vi "FTW-CSV-Variant-Traverse-Array.vi"(0 "Variant":variant, 1 "Options":T1={"String Quotes"=FALSE, "Real Format"="%#_15g", "Timestamp Format"="%^<%Y-%m-%dT%H:%M:%S%3uZ>T", "Delimiter"=","}, 11 "error in":errorcluster) -> (4 "CSV String":string, 15 "error out":errorcluster)   [LabVIEW 2015]
uses:
  FTW-CSV-SerializeOptions.ctl
  <vilib>/Utility/Data Type/NI_Data Type.lvlib
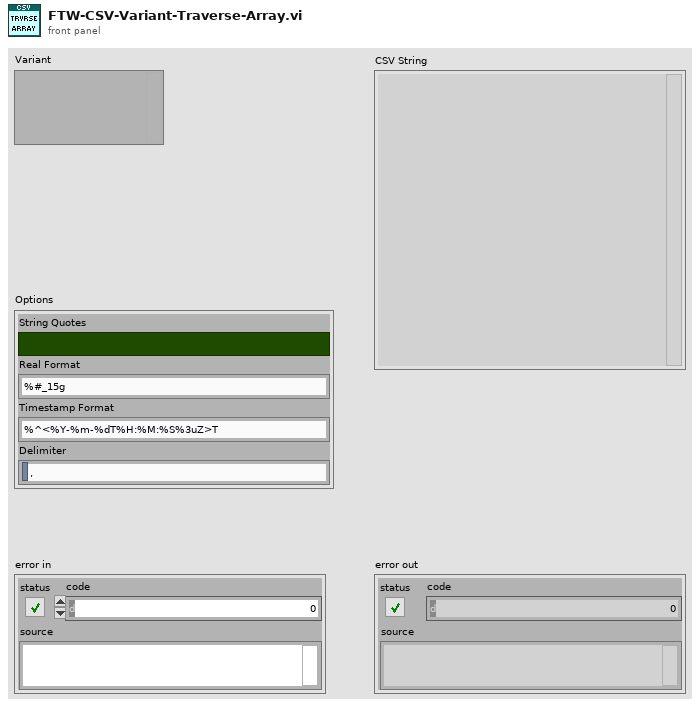
[diagram p1: front panel]
types:
  T1 = typedef "FTW-CSV-SerializeOptions.ctl" = cluster{"String Quotes":bool, "Real Format":string, "Timestamp Format":string, "Delimiter":string}
  T2 = typedef "NI_Data Type.lvlib/Data Type.ctl" = enum8{"Invalid Type", "Void", "I8", "I16", "I32", "I64", "U8", "U16", "U32", "U64", "Single Float", "Double Float", "Extended Float", "Single Complex", "Double Complex", "Extended Complex", "Enum U8", "Enum U16", "Enum U32", "Enum U64", "Single Float With Unit", "Double Float With Unit", "Extended Float With Unit", "Single Complex with Unit", "Double Complex with Unit", "Extended Complex with Unit", "Boolean", "String", "Path", "Picture", "Tag", "Array", "Cluster", "Variant", "LV Variant", "Waveform", "Timestamp", "Digital Waveform", "Digital Data", "ExpressData", "Refnum", "External Data", "VI", "Poly VI", "LabVIEW Class Instance", "Fixed Point"}
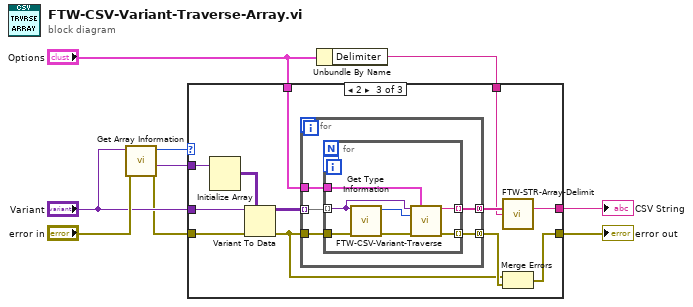
[diagram p0: block diagram]
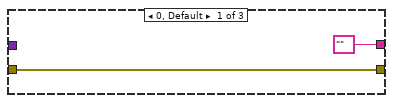
[diagram p2: hidden frame]
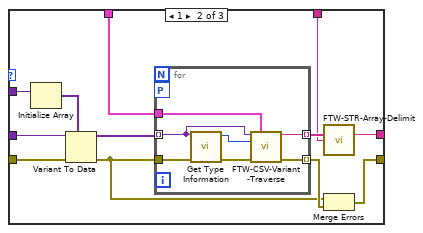
[diagram p3: hidden frame]
diagram:
  n1 = call <vilib>:"Get Array Information.vi"("error in (no error)"="error in", "Variant"="Variant") -> ("error out"=w4:errorcluster, "Array Element Data Type"=w2:variant, "Number of Dimensions"=w3:i32)  [unwired: 6 in, 1 out]
  n2 = Unbundle By Name("Options") -> ("Delimiter"=w1:string)
  n3 = case shown="2" w3 {
    tunnel: [w11 w15 w34] -> w8
    tunnel: w4 -> [w11 w22 w41]
    tunnel: w2 -> [_ w18 w37]
    tunnel: ["" ("empty string") w20 w39] -> w7
    tunnel: "Variant" -> [_ w19 w38]
    tunnel: "Options" -> [_ w13 w32]
    tunnel: w1 -> [_ w12 w31]
    frame 0, Default {
    }
    frame 1 {
      n4 = Initialize Array(w18) -> (w17:variant[])  [unwired: 1 in]
      n5 = Variant To Data(error in=w22, type=w17, Variant=w19) -> (data=w16:variant[], error out=w14:errorcluster)
      n6 = for {
        tunnel: w16 -> [w25] mode=indexing
        tunnel: [w29] -> w21 mode=indexing
        tunnel: w14 -> [w28]
        tunnel: [w30] -> w23 mode=indexing
        tunnel: w13 -> [w27]
        workers-P: _ -> [_]
        n7 = call <vilib>:"Get Type Information.vi"("error in (no error)"=w28, "Variant"=w25) -> ("error out"=w26:errorcluster, "Type"=w24:T2)  [unwired: 5 in, 3 out]
        n8 = call "FTW-CSV-Variant-Traverse.vi"("Variant"=w25, "Options"=w27, "Type"=w24, "error in"=w26) -> ("CSV String"=w29:string, "error out"=w30:errorcluster)  [unwired: 10 in]
      }
      n9 = call "FTW-STR-Array-Delimit.vi"("Array of Strings"=w21, "Delimiter"=w12) -> ("Delimited String"=w20:string)  [unwired: 13 in]
      n10 = Merge Errors(w14, w23) -> (w15:errorcluster)
    }
    frame 2 {
      n11 = Initialize Array(w37) -> (w36:variant[][])  [unwired: 2 in]
      n12 = Variant To Data(error in=w41, type=w36, Variant=w38) -> (data=w35:variant[][], error out=w33:errorcluster)
      n13 = for {
        tunnel: [w47] -> w42 mode=concatenating
        tunnel: [w46] -> w40 mode=concatenating
        tunnel: w35 -> [w45] mode=indexing
        tunnel: w33 -> [w44]
        tunnel: w32 -> [w43]
        n14 = for {
          tunnel: w45 -> [w49] mode=indexing
          tunnel: [w53] -> w46 mode=indexing
          tunnel: w44 -> [w52]
          tunnel: [w54] -> w47 mode=indexing
          tunnel: w43 -> [w51]
          workers-P: _ -> [_]
          n15 = call <vilib>:"Get Type Information.vi"("error in (no error)"=w52, "Variant"=w49) -> ("error out"=w50:errorcluster, "Type"=w48:T2)  [unwired: 5 in, 3 out]
          n16 = call "FTW-CSV-Variant-Traverse.vi"("Variant"=w49, "Options"=w51, "Type"=w48, "error in"=w50) -> ("CSV String"=w53:string, "error out"=w54:errorcluster)  [unwired: 10 in]
        }
      }
      n17 = call "FTW-STR-Array-Delimit.vi"("Array of Strings"=w40, "Delimiter"=w31) -> ("Delimited String"=w39:string)  [unwired: 13 in]
      n18 = Merge Errors(w33, w42) -> (w34:errorcluster)
    }
  }
  "error out" <- w8
  "CSV String" <- w7
